vi "lv.vi"() -> ()   [LabVIEW 2014]
uses:
  LabVIEW.exe
panel:
  out "Cursor":i32
  in  "Console":string
  in  "Run":bool
  in  "Task":string(combo)="test"
  in  "Quit":bool
  in  "File":path
  in  "Engine":enum16{"luajit", "lua53"}(ring)=enum."lua53"
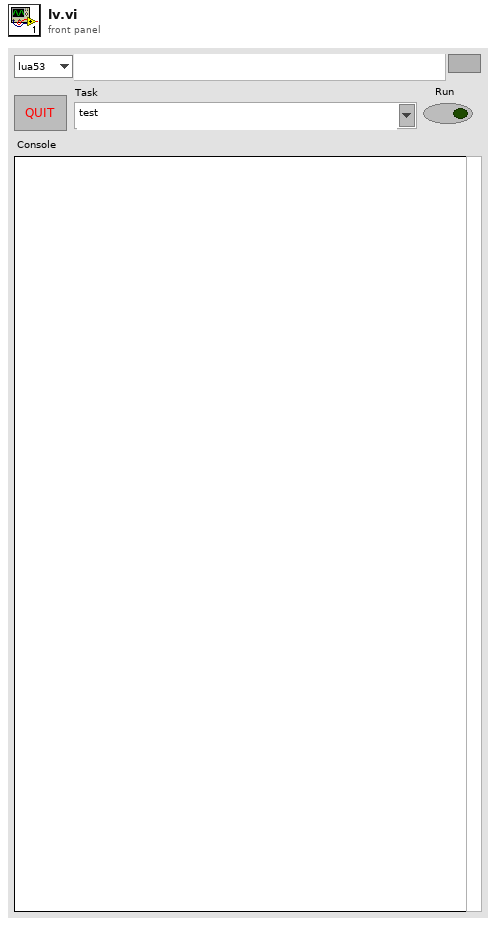
[diagram p1: front panel]
types:
  T1 = typedef "eventvkey.ctl" = enum16{"ASCII", "Enter", "Return", "Shift", "Ctrl", "Alt", "Cmd", "Opt", "Caps", "NumLock", "Clear", "Break", "Up", "Down", "Left", "Right", "Insert", "Delete", "Home", "End", "PageUp", "PageDown", "Escape", "Help", "Pause", "ScrollLock", "F1", "F2", "F3", "F4", "F5", "F6", "F7", "F8", "F9", "F10", "F11", "F12", "F13", "F14", "F15", "F16", "F17", "F18", "F19", "F20", "F21", "F22", "F23", "F24", "Play", "VolumeUp", "VolumeDown", "Mute", "Two Byte Char"}
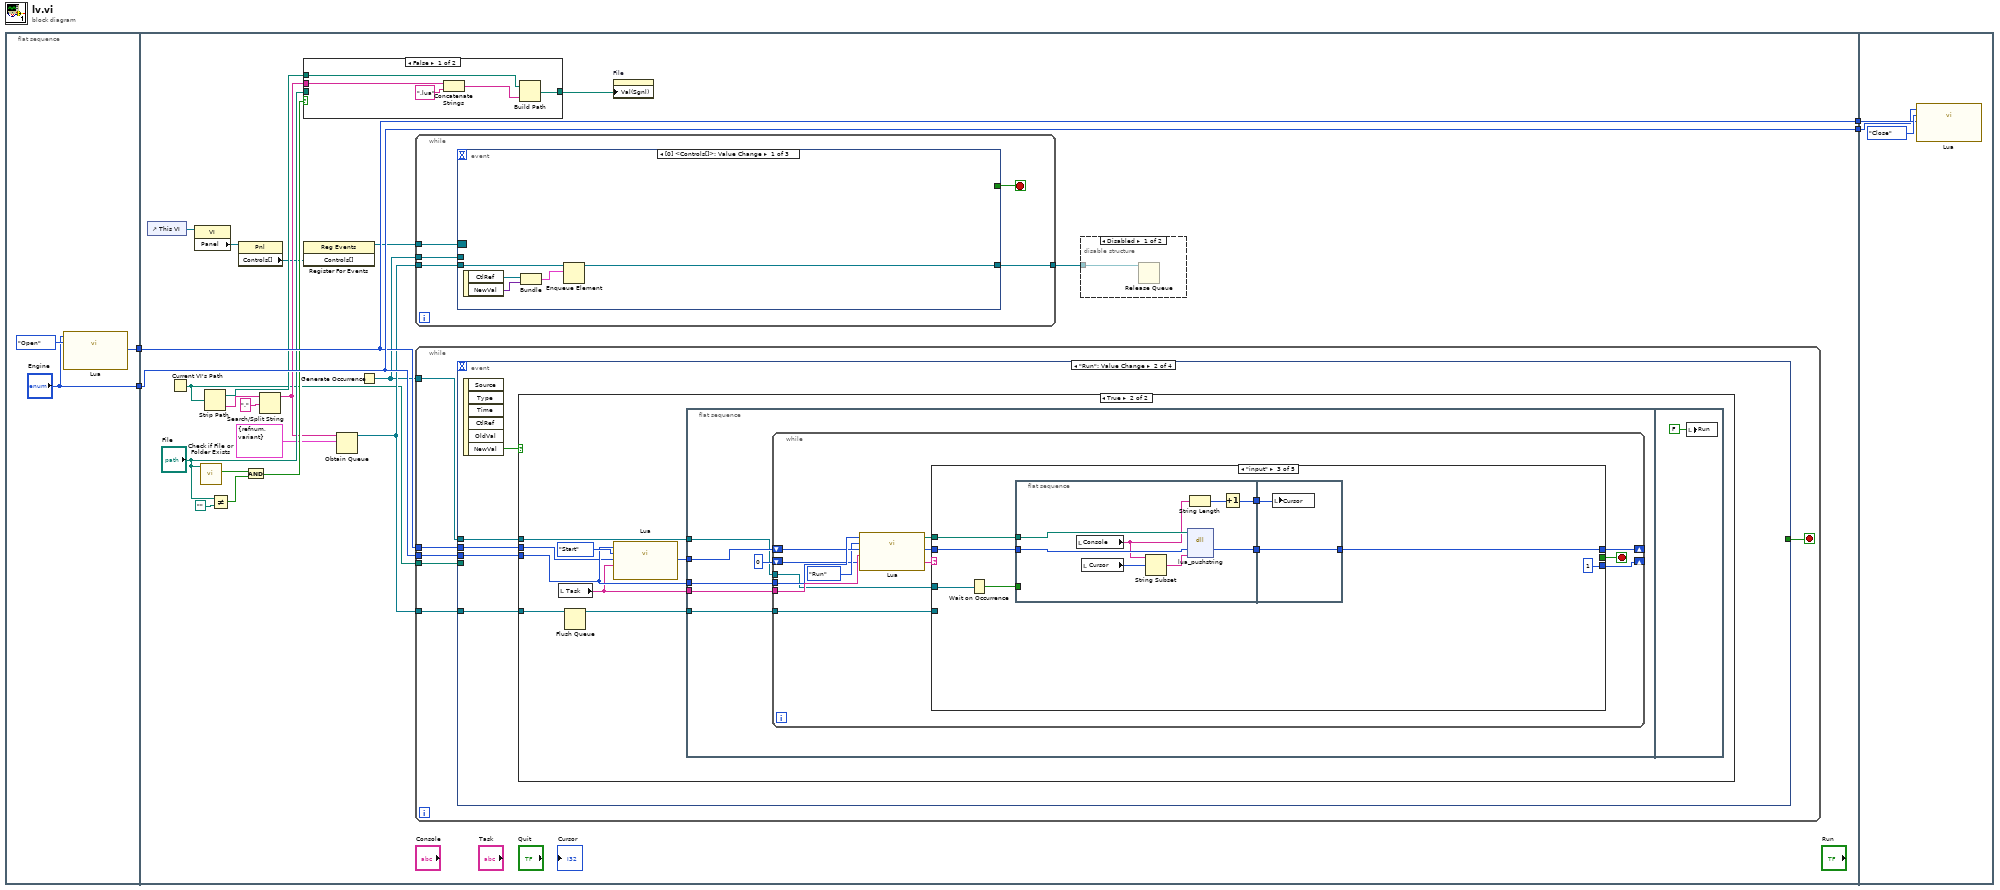
[diagram p0: block diagram]
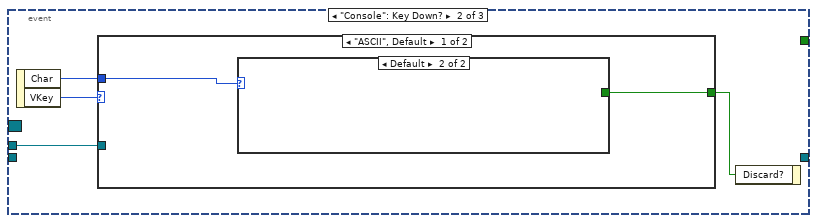
[diagram p3: hidden frame]
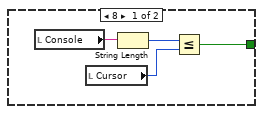
[diagram p4: hidden frame]
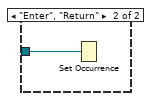
[diagram p5: hidden frame]
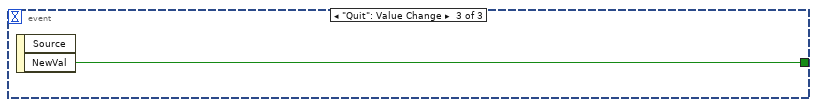
[diagram p6: hidden frame]
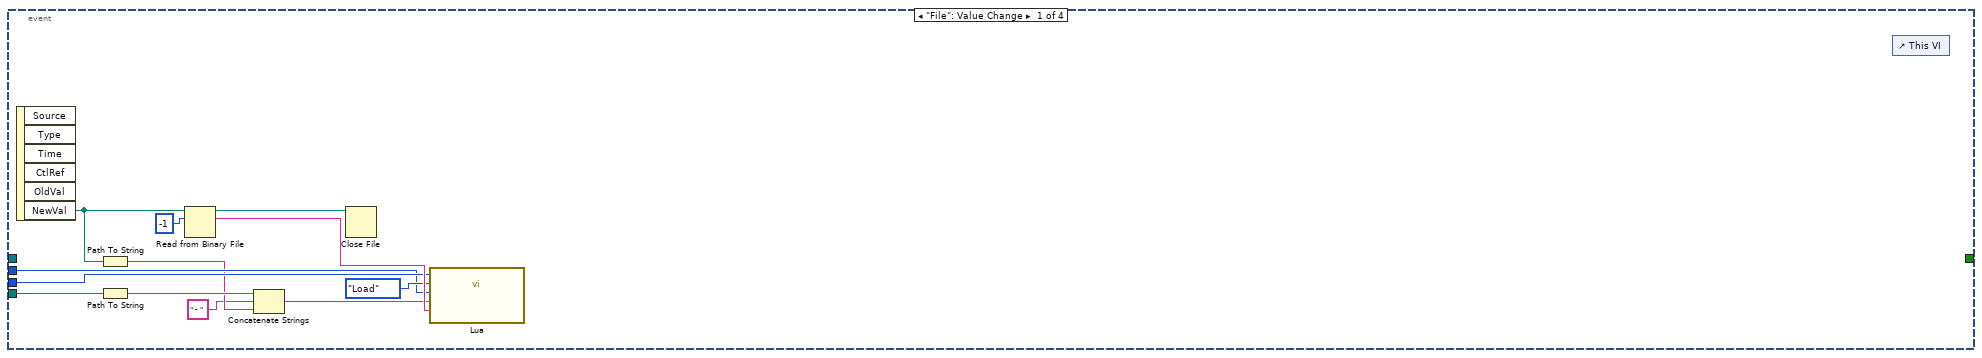
[diagram p8: hidden frame]
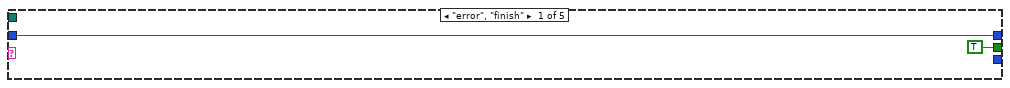
[diagram p10: hidden frame]
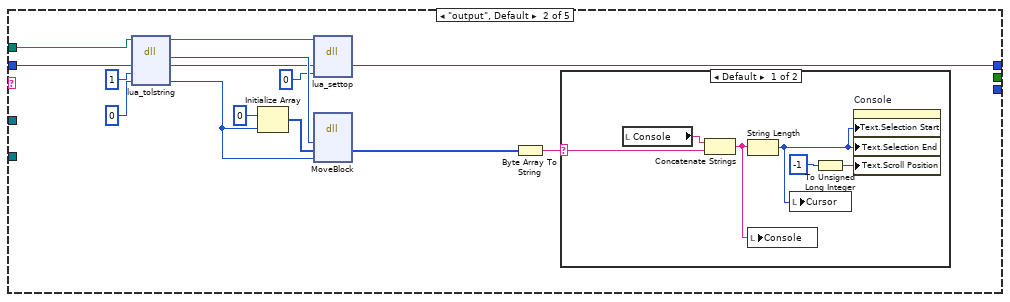
[diagram p11: hidden frame]
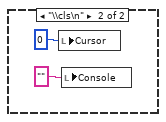
[diagram p12: hidden frame]
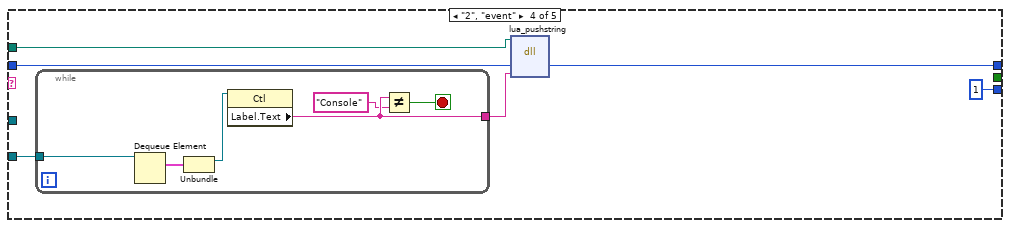
[diagram p13: hidden frame]
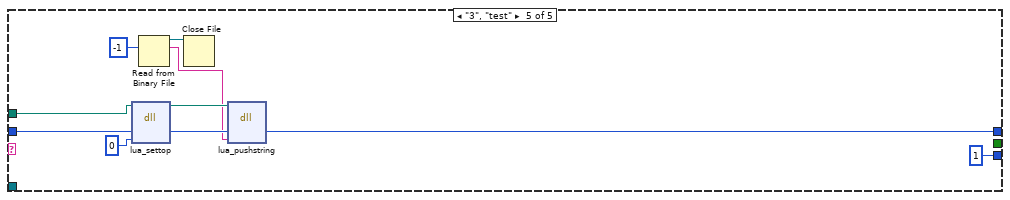
[diagram p14: hidden frame]
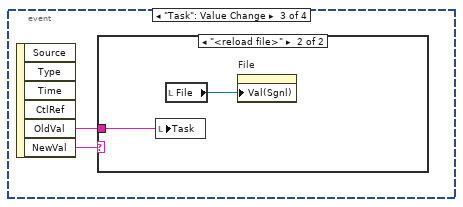
[diagram p15: hidden frame]
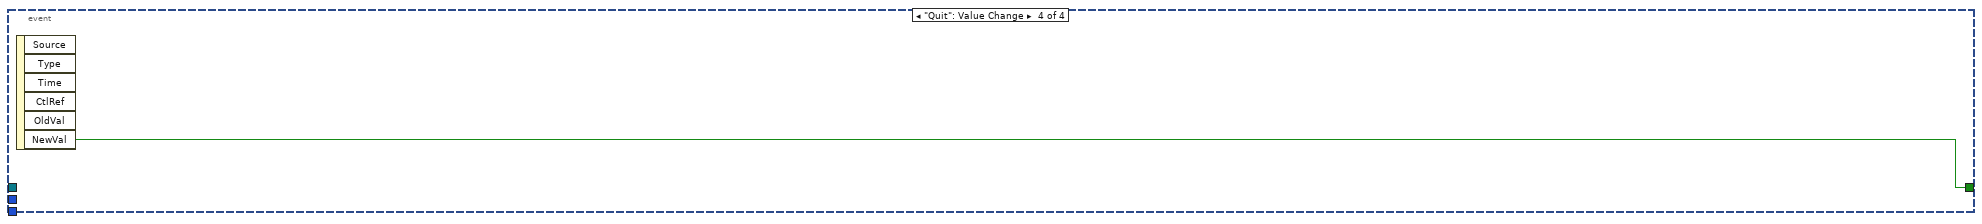
[diagram p17: hidden frame]
diagram:
  n1 = flat-sequence {
    tunnel: ["Engine"] -> w2
    tunnel: [w5] -> w1
    tunnel: [w27] -> w4
    tunnel: [w28] -> w3
    tunnel: w2 -> [w28]
    tunnel: w1 -> [w27]
    tunnel: w4 -> [w179]
    tunnel: w3 -> [w178]
    frame #0 {
      n2 = call "Lua.vi"("Lua Version"="Engine", "Action"=enum16{"Open", "Load", "Start", "Run", "Close"}."Open") -> ("L Out"=w5:u64)  [unwired: 3 in, 2 out]
    }
    frame #1 {
      n3 = control-ref of="This VI"() -> (w13:refnum<vi>)
      n4 = Current VI's Path() -> (path=w9:path)
      n5 = property class="VI"(reference=w13) -> ("Panel"=w14:refnum<vi>)  [unwired: 1 in, 2 out]
      n6 = call <vilib>:"Check if File or Folder Exists.vi"("path"="File") -> ("file or folder exists?"=w25:bool)  [unwired: 8 in, 2 out]
      n7 = Strip Path(path=w9) -> (stripped path=w18:path, name=w19:string)
      n8 = Not Equal?(x="File", y=path "") -> (x != y?=w24:bool)
      n9 = property class="Pnl"(reference=w14) -> ("Controls[]"=w12:refnum<vi>[])  [unwired: 1 in, 2 out]
      n10 = And(x=w25, y=w24) -> (x .and. y?=w26:bool)
      n11 = Search/Split String(string=w19, search string/char (-)=".") -> (substring before match=w15:string)  [unwired: 1 in, 2 out]
      n12 = case shown="False" w26 {
        tunnel: [w54 w57] -> w21
        tunnel: "File" -> [_ w57]
        tunnel: w15 -> [w53 _]
        tunnel: w18 -> [w52 _]
        frame False {
          n13 = Concatenate Strings(w53, ".lua" ("string")) -> (w56:string)
          n14 = Build Path(base path=w52, name or relative path=w56) -> (appended path=w54:path)
        }
        frame True {
        }
      }
      n15 = register-events(w12) -> (reference out=w17:refnum<event-registration>)  [unwired: 2 in, 1 out]
      n16 = Obtain Queue(name (unnamed)=w15, element data type=cluster{"CtlRef":refnum<vi>, "NewVal":variant} {"CtlRef"=refnum, "NewVal"=variant} ("output cluster")) -> (queue out=w11:refnum<queue>)  [unwired: 3 in, 2 out]
      n17 = Generate Occurrence() -> (w8:refnum<k4>)
      n18 = while {
        tunnel: w11 -> [w34]
        tunnel: w17 -> [w33]
        tunnel: [w32] -> w16
        tunnel: w8 -> [w30]
        stop <- w31 stop-if-true
        n19 = event shown="[0] <Controls[]>: Value Change" {
          selector: w33 -> [_ _ _]
          dyn-events: _ -> [_ _ _]
          timeout: _ -> [_ _ _]
          tunnel: w34 -> [w39 _ _]
          tunnel: [w36 _ _] -> w32
          tunnel: [_ _ w51] -> w31
          tunnel: w30 -> [_ w42 _]
          event Value Change {
            n20 = event-data() -> ("CtlRef"=w35:refnum<vi>, "NewVal"=w38:variant)  [unwired: 1 in]
            n21 = Bundle("CtlRef"=w35, "NewVal"=w38) -> (w37:cluster{"CtlRef":refnum<vi>, "NewVal":variant})  [unwired: 1 in]
            n22 = Enqueue Element(queue=w39, element=w37) -> (queue out=w36:refnum<queue>)  [unwired: 2 in, 2 out]
          }
          event "Console": Key Down? {
            n23 = event-data() -> ("Char"=w41:i16, "VKey"=w43:T1)  [unwired: 1 in]
            n24 = case shown="\"ASCII\", Default" w43 {
              tunnel: w42 -> [_ w50]
              tunnel: w41 -> [w45 _]
              tunnel: [w44 _] -> w40
              frame "ASCII", Default {
                n25 = case shown="Default" w45 {
                  tunnel: [w46 _] -> w44
                  frame 8 {
                    n26 = local read "Console"() -> (w49:string)
                    n27 = local read "Cursor"() -> (w47:i32)
                    n28 = String Length(string=w49) -> (length=w48:i32)
                    n29 = Less Or Equal?(x=w48, y=w47) -> (x <= y?=w46:bool)
                  }
                  frame Default {
                  }
                }
              }
              frame "Enter", "Return" {
                n30 = Set Occurrence(w50) -> ()
              }
            }
            n31 = event-data("Discard?"=w40) -> ()  [unwired: 1 in, 1 out]
          }
          event "Quit": Value Change {
            n32 = event-data() -> ("NewVal"=w51:bool)  [unwired: 1 in, 1 out]
          }
        }
      }
      n33 = while {
        tunnel: w28 -> [w63]
        tunnel: w27 -> [w62]
        tunnel: w11 -> [w60]
        tunnel: w9 -> [w59]
        tunnel: w8 -> [w58]
        stop <- w61 stop-if-true
        n34 = event shown="[1] \"Run\": Value Change" {
          selector: _ -> [_ _ _ _]
          dyn-events: _ -> [_ _ _ _]
          timeout: _ -> [_ _ _ _]
          tunnel: w63 -> [w71 w79 _ _]
          tunnel: w62 -> [w70 w78 _ _]
          tunnel: [_ _ _ w177] -> w61
          tunnel: w60 -> [_ w77 _ _]
          tunnel: w59 -> [w68 _ _ _]
          tunnel: w58 -> [_ w76 _ _]
          event "File": Value Change {
            n35 = event-data() -> ("NewVal"=w69:path)  [unwired: 1 in, 5 out]
            n36 = Path To String(path=w69) -> (string=w66:string)
            n37 = Path To String(path=w68) -> (string=w67:string)
            n38 = Read from Binary File(10:-1 ("count (1)"), 11:w69) -> (2:w75:string, 3:w74:refnum<file>)  [unwired: 4 in, 2 out]
            n39 = Concatenate Strings(w67, " - " ("string"), w66) -> (w64:string)
            n40 = Close File(refnum=w74) -> ()  [unwired: 1 in, 2 out]
            n41 = call "Lua.vi"("Lua Version"=w71, "Action"=enum16{"Open", "Load", "Start", "Run", "Close"}."Load", "L In"=w70, "Name"=w64, "Arg"=w75) -> ()  [unwired: 3 out]
            n42 = control-ref of="This VI"() -> ()  [unwired: 1 out]
          }
          event "Run": Value Change {
            n43 = event-data() -> ("NewVal"=w80:bool)  [unwired: 1 in, 5 out]
            n44 = case shown="True" w80 {
              tunnel: w79 -> [_ w86]
              tunnel: w78 -> [_ w85]
              tunnel: w77 -> [_ w83]
              tunnel: w76 -> [_ w81]
              frame False {
              }
              frame True {
                n45 = local read "Task"() -> (w84:string)
                n46 = Flush Queue(queue=w83) -> (queue out=w82:refnum<queue>)  [unwired: 1 in, 2 out]
                n47 = call "Lua.vi"("Lua Version"=w86, "Action"=enum16{"Open", "Load", "Start", "Run", "Close"}."Start", "L In"=w85, "Name"=w84) -> ("L Out"=w87:u64)  [unwired: 1 in, 2 out]
                n48 = flat-sequence {
                  tunnel: w84 -> [w94]
                  tunnel: w87 -> [w92]
                  tunnel: w86 -> [w91]
                  tunnel: w82 -> [w90]
                  tunnel: w81 -> [w89]
                  frame #0 {
                    n49 = while {
                      tunnel: w94 -> [w107]
                      tunnel: w91 -> [w106]
                      shift-right: [w99] -> _
                      shift-left: w92 -> [w105]
                      shift-right: [w100] -> _
                      shift-left: 0 ("int") -> [w101]
                      tunnel: w90 -> [w96]
                      tunnel: w89 -> [w95]
                      stop <- w102 stop-if-true
                      n50 = call "Lua.vi"("Lua Version"=w106, "Action"=enum16{"Open", "Load", "Start", "Run", "Close"}."Run", "L In"=w105, "Name"=w107, "Arg"=w101) -> ("Lua Dll"=w97:path, "L Out"=w98:u64, "Status"=w103:string)
                      n51 = case shown="\"input\"" w103 {
                        tunnel: [TRUE _ _ _ _] -> w102
                        tunnel: [_ _ 1 ("int") 1 ("int") 1 ("int")] -> w100
                        tunnel: w98 -> [w108 w113 w138 w153 w168]
                        tunnel: [w108 w112 w137 w151 w163] -> w99
                        tunnel: w97 -> [_ w114 w139 w152 w169]
                        tunnel: w96 -> [_ _ _ w155 _]
                        tunnel: w95 -> [_ _ w134 _ _]
                        frame "error", "finish" {
                        }
                        frame "output", Default {
                          n52 = dll-call lib="lua5.dll" fn="lua_tolstring"(path in=w114, "L"=w113, "idx"=1, "len"=0) -> (path out=w116:path, "str"=w121:u64, "L"=w117:u64, "len"=w119:i32)  [unwired: 3 in, 1 out]
                          n53 = Initialize Array(u8 0 ("element"), w119) -> (w120:u8[])
                          n54 = dll-call lib="lua5.dll" fn="lua_settop"(path in=w116, "L"=w117, "idx"=0) -> ("L"=w112:u64)  [unwired: 4 in, 2 out]
                          n55 = dll-call lib="LabVIEW.exe" fn="MoveBlock"("src"=w121, "dest"=w120, "size"=w119) -> ("dest"=w111:u8[])  [unwired: 6 in, 2 out]
                          n56 = Byte Array To String(unsigned byte array=w111) -> (string=w110:string)
                          n57 = case shown="Default" w110 {
                            selector: w110 -> [w129 _]
                            frame Default {
                              n58 = local read "Console"() -> (w128:string)
                              n59 = Concatenate Strings(w128, w129) -> (w127:string)
                              n60 = String Length(string=w127) -> (length=w126:i32)
                              n61 = local write "Console"(w127) -> ()
                              n62 = local write "Cursor"(w126) -> ()
                              n63 = To Unsigned Long Integer(number=-1 ("Text.Scroll Position")) -> (unsigned 32bit integer=w125:u32)
                              n64 = property on="Console" class="Str"("Text.Selection Start"=w126, "Text.Selection End"=w126, "Text.Scroll Position"=w125) -> ()  [unwired: 2 in, 2 out]
                            }
                            frame "\\cls\n" {
                              n65 = local write "Cursor"(0 ("Cursor")) -> ()
                              n66 = local write "Console"("" ("Output")) -> ()
                            }
                          }
                        }
                        frame "input" {
                          n67 = Wait on Occurrence(2:w134) -> (0:w135:bool)  [unwired: 2 in]
                          n68 = flat-sequence {
                            tunnel: w139 -> [w147]
                            tunnel: w138 -> [w146]
                            tunnel: w135 -> [_]
                            tunnel: [w145] -> w133
                            tunnel: [w140] -> w132
                            tunnel: [w149] -> w137
                            tunnel: w133 -> [w149]
                            tunnel: w132 -> [w148]
                            frame #0 {
                              n69 = local read "Console"() -> (w142:string)
                              n70 = local read "Cursor"() -> (w144:i32)
                              n71 = String Subset(string=w142, offset (0)=w144) -> (substring=w143:string)  [unwired: 1 in]
                              n72 = dll-call lib="lua5.dll" fn="lua_pushstring"(path in=w147, "L"=w146, "n"=w143) -> ("L"=w145:u64)  [unwired: 4 in, 2 out]
                              n73 = String Length(string=w142) -> (length=w141:i32)
                              n74 = Increment(x=w141) -> (x+1=w140:i32)
                            }
                            frame #1 {
                              n75 = local write "Cursor"(w148) -> ()
                            }
                          }
                        }
                        frame "2", "event" {
                          n76 = while {
                            tunnel: w155 -> [w161]
                            tunnel: [w158] -> w154
                            stop <- w156 stop-if-true
                            n77 = Dequeue Element(queue=w161) -> (element=w160:cluster{"CtlRef":refnum<vi>, "NewVal":variant})  [unwired: 2 in, 3 out]
                            n78 = Unbundle(w160) -> ("CtlRef"=w159:refnum<vi>)  [unwired: 1 out]
                            n79 = property class="Ctl"(reference=w159) -> ("Label.Text"=w158:string)  [unwired: 1 in, 2 out]
                            n80 = Not Equal?(x=w158, y="Console") -> (x != y?=w156:bool)
                          }
                          n81 = dll-call lib="lua5.dll" fn="lua_pushstring"(path in=w152, "L"=w153, "n"=w154) -> ("L"=w151:u64)  [unwired: 4 in, 2 out]
                        }
                        frame "3", "test" {
                          n82 = dll-call lib="lua5.dll" fn="lua_settop"(path in=w169, "L"=w168, "idx"=0) -> (path out=w166:path, "L"=w165:u64)  [unwired: 4 in, 1 out]
                          n83 = Read from Binary File(10:-1 ("count (1)")) -> (2:w164:string, 3:w170:refnum<file>)  [unwired: 5 in, 2 out]
                          n84 = Close File(refnum=w170) -> ()  [unwired: 1 in, 2 out]
                          n85 = dll-call lib="lua5.dll" fn="lua_pushstring"(path in=w166, "L"=w165, "n"=w164) -> ("L"=w163:u64)  [unwired: 4 in, 2 out]
                        }
                      }
                    }
                  }
                  frame #1 {
                    n86 = local write "Run"(FALSE ("Run")) -> ()
                  }
                }
              }
            }
          }
          event "Task": Value Change {
            n87 = event-data() -> ("OldVal"=w173:string, "NewVal"=w174:string)  [unwired: 1 in, 4 out]
            n88 = case shown="\"<reload file>\"" w174 {
              tunnel: w173 -> [_ w175]
              frame "False", Default {
              }
              frame "<reload file>" {
                n89 = local write "Task"(w175) -> ()
                n90 = local read "File"() -> (w176:path)
                n91 = property on="File" class="Path"("Val(Sgnl)"=w176) -> ()  [unwired: 2 in, 2 out]
              }
            }
          }
          event "Quit": Value Change {
            n92 = event-data() -> ("NewVal"=w177:bool)  [unwired: 1 in, 5 out]
          }
        }
      }
      n93 = property on="File" class="Path"("Val(Sgnl)"=w21) -> ()  [unwired: 2 in, 2 out]
      n94 = disable-structure shown="Disabled" {
        disable-tunnel: w16 -> [w29 _]
        frame Disabled {
          n95 = Release Queue(queue=w29) -> ()  [unwired: 2 in, 3 out]
        }
        frame Enabled {
        }
      }
    }
    frame #2 {
      n96 = call "Lua.vi"("Lua Version"=w178, "Action"=enum16{"Open", "Load", "Start", "Run", "Close"}."Close", "L In"=w179) -> ()  [unwired: 2 in, 3 out]
    }
  }
